vi "Update Results.vi"(8 "error in (no error)":errorcluster, 10 "Measurement Results":variant, 11 "MeasurementContext in":refnum<class "Measure Call Context.lvclass">) -> (0 "error out":errorcluster, 3 "MeasurementContext out":refnum<class "Measure Call Context.lvclass">)   [LabVIEW 2020, in "MeasurementLink Measurement Server.lvlib" / "Measure Call Context.lvclass"]
doc: "Sends measurement updates to a measurement client, like InstrumentStudio. Do not use this VI to write the final results. Instead, use the Measurement Results indicator of the Measurement Logic VI to write the final measurement result.\n\nThis VI must be called with the Measurement Results cluster as the input. You must always update all elements of the cluster, including unchanged values.\n\nInstrumentStudio does not cache data from previous updates so you must write all of the data to the cluster to display cumulative updates.\n\nTestStand gnores updates from this VI and only uses the final measurement result."
uses:
  Measure Call Context.lvclass
  Classes/IMeasurementService/IMeasurementService.lvclass
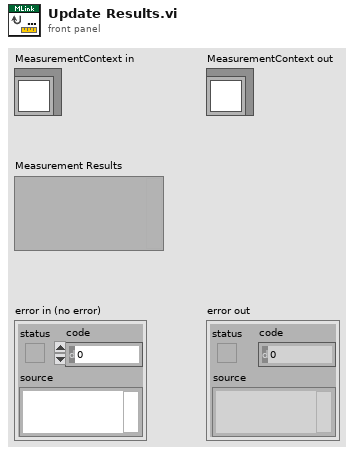
[diagram p1: front panel]
types:
  T1 = typedef "MeasurementLink Measurement Server.lvlib/MeasurementContext.lvclass/Data.ctl" = cluster{"PinMapContext":T2, "gRPCServerId":T3, "IMeasurementService":refnum<class "IMeasurementService.lvclass">, "MeasurementPluginService":refnum<class "Measurement Plugin Service.lvclass">, "reserved session infos":set{T4}}
  T2 = typedef "MeasurementLink Measurement Server.lvlib/PinMapContext.ctl" = cluster{"pin_map_id":string, "sites":i32[]}
  T3 = typedef "grpc-lvsupport-release.lvlib/grpcId.ctl" = u64
  T4 = typedef "MeasurementLink Session Management Client.lvlib/ni_measurementlink_sessionmanagement_v1_SessionInformation.ctl" = cluster{"session":T5, "resource_name":string, "channel_list":string, "instrument_type_id":string, "session_exists":bool, "channel_mappings":T6[]}
  T5 = typedef "MeasurementLink Session Management Client.lvlib/nidevice_grpc_Session.ctl" = cluster{"name":string}
  T6 = typedef "MeasurementLink Session Management Client.lvlib/ni_measurementlink_sessionmanagement_v1_ChannelMapping.ctl" = cluster{"pin_or_relay_name":string, "site":i32, "channel":string}
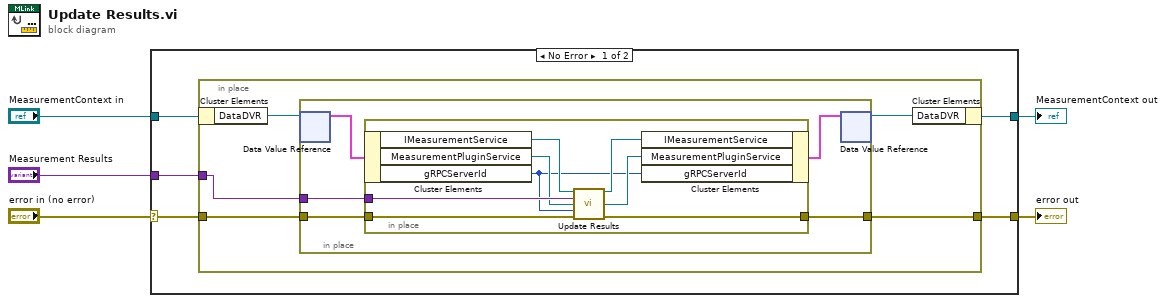
[diagram p0: block diagram]
diagram:
  n1 = case shown="No Error" "error in (no error)" {
    selector: "error in (no error)" -> [w8 w30]
    tunnel: [w7 w30] -> w4
    tunnel: [w6 w29] -> w2
    tunnel: "MeasurementContext in" -> [w10 w29]
    tunnel: "Measurement Results" -> [w9 _]
    frame No Error {
      n2 = in-place {
        in-place-border: w9 -> [w15]
        in-place-border: w8 -> [w14]
        in-place-border: [w13] -> w7
        n3 = in-place-cluster #1(w10) -> ("DataDVR"=w12:refnum<data-value>)
        n4 = in-place {
          in-place-border: w15 -> [w20]
          in-place-border: w14 -> [w19]
          in-place-border: [w18] -> w13
          n5 = in-place-dvr #2(w12) -> (w17:T1)  [unwired: 1 out]
          n6 = in-place {
            in-place-border: w20 -> [w28]
            in-place-border: w19 -> [w27]
            in-place-border: [w26] -> w18
            n7 = in-place-cluster #3(w17) -> ("IMeasurementService"=w25:refnum<class "IMeasurementService.lvclass">, "MeasurementPluginService"=w24:refnum<class "Measurement Plugin Service.lvclass">, "gRPCServerId"=w21:T3)
            n8 = call-dynamic "Update Results.vi"("IMeasurementService in"=w25, "Measurement Results"=w28, "MeasurementPluginService in"=w24, "gRPCid in"=w21, "error in (no error)"=w27) -> ("IMeasurementService out"=w23:refnum<class "IMeasurementService.lvclass">, "MeasurementPluginService out"=w22:refnum<class "Measurement Plugin Service.lvclass">, "error out"=w26:errorcluster)  [unwired: 8 in]
            n9 = in-place-cluster #3("IMeasurementService"=w23, "MeasurementPluginService"=w22, "gRPCServerId"=w21) -> (w16:T1)
          }
          n10 = in-place-dvr #2(w16) -> (w11:refnum<data-value>)  [unwired: 1 out]
        }
        n11 = in-place-cluster #1("DataDVR"=w11) -> (w6:refnum<class "Measure Call Context.lvclass">)
      }
    }
    frame Error {
    }
  }
  "error out" <- w4
  "MeasurementContext out" <- w2
